vi "svx_Colormap Num to String.vi"(7 "Unit":string="X", 11 "Order":dbl) -> (3 "String":string, 4 "Integer":bool)   [LabVIEW 2017, in "SVX Colormap.xctl"]
uses:
  <vilib>/addons/_XControls/Colormap/SVX Colormap.xctl
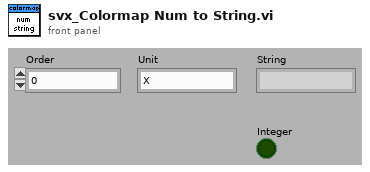
[diagram p1: front panel]
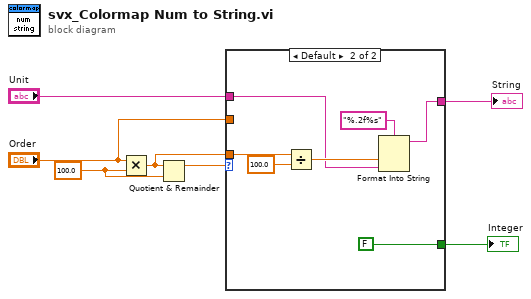
[diagram p0: block diagram]
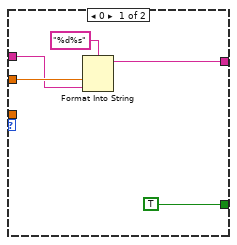
[diagram p2: hidden frame]
diagram:
  w7 = 100.0 ("y")
  n1 = Multiply(x="Order", y=w7) -> (x*y=w4:dbl)
  n2 = Quotient & Remainder(x=w4, y=w7) -> (x-y*floor(x/y)=w6:dbl)  [unwired: 1 out]
  n3 = case shown="Default" w6 {
    tunnel: "Order" -> [w11 _]
    tunnel: w4 -> [_ w19]
    tunnel: [w10 w15] -> w3
    tunnel: [TRUE FALSE] -> w2
    tunnel: "Unit" -> [w8 w13]
    frame 0 {
      n4 = Format Into String(format string="%d%s", w11, w8) -> (resulting string=w10:string)  [unwired: 2 in, 1 out]
    }
    frame Default {
      n5 = Divide(x=w19, y=100.0) -> (x/y=w16:dbl)
      n6 = Format Into String(format string="%.2f%s", w16, w13) -> (resulting string=w15:string)  [unwired: 2 in, 1 out]
    }
  }
  "String" <- w3
  "Integer" <- w2
